vi "analyze anal files.vi"() -> ()   [LabVIEW 2024]
panel:
  out "z":cluster{dbl[], dbl[]}[](graph)=[{[-3.1923908912798504, -2.9876019813869705, -2.782813071494091, -2.578024161601211, -2.3732352517083317, -2.1684463418154523, -1.9636574319225724, -1.7588685220296927, -1.554079612136813, -1.3492907022439335, -1.1445017923510539, -0.9397128824581742, -0.7349239725652945, -0.5301350626724148, -0.3253461527795352, -0.12055724288665554, 0.08423166700622411, 0.28902057689910376, 0.4938094867919834, 0.698598396684863, 0.9033873065777427, 1.1081762164706224, 1.312965126363502, 1.5177540362563817, 1.7225429461492614, 1.9273318560421409, 2.1321207659350208, 2.3369096758279, 2.54169858572078, 2.7464874956136596], [9.0, 17.0, 27.0, 32.0, 37.0, 44.0, 46.0, 48.0, 62.0, 79.0, 99.0, 123.0, 154.0, 201.0, 258.0, 267.0, 252.0, 248.0, 225.0, 186.0, 138.0, 99.0, 66.0, 47.0, 34.0, 20.0, 11.0, 8.0, 4.0, 1.0]}, {array[1000 elements], array[1000 elements]}]
  out "y":cluster{dbl[], dbl[]}[](graph)=[{[-1.5308237164517153, -1.3260348065588357, -1.121245896665956, -0.9164569867730764, -0.7116680768801967, -0.506879166987317, -0.30209025709443743, -0.09730134720155777, 0.10748756269132188, 0.31227647258420155, 0.5170653824770812, 0.7218542923699608, 0.9266432022628405, 1.13143211215572, 1.3362210220485997], [0.0, 11.0, 10.0, 11.0, 9.0, 20.0, 83.0, 267.0, 252.0, 84.0, 27.0, 20.0, 17.0, 32.0, 17.0]}, {array[1000 elements], array[1000 elements]}]
  out "x":cluster{dbl[], dbl[]}[](graph)=[{[-1.8188204016021599, -1.6140314917092802, -1.4092425818164007, -1.204453671923521, -0.9996647620306414, -0.7948758521377617, -0.590086942244882, -0.3852980323520024, -0.1805091224591227, 0.024279787433756934, 0.2290686973266366, 0.4338576072195162, 0.6386465171123958, 0.8434354270052755, 1.0482243368981552, 1.2530132467910349, 1.4578021566839146, 1.6625910665767942], [18.0, 17.0, 18.0, 25.0, 36.0, 54.0, 98.0, 171.0, 230.0, 267.0, 219.0, 145.0, 83.0, 62.0, 52.0, 34.0, 33.0, 33.0]}, {array[1000 elements], array[1000 elements]}]
  in  "z length":i32=15
  in  "index (row) 2":i32=10
  in  "disabled index (col)":i32=10
  in  "index (row)":i32=10
  out "Waveform Graph":u16[][](graph)=[[119, 118, 117, 118, 125, 136, 154, 198, 271, 330, 367, 319, 245, 183, 162, 152, 134, 133, 133, 131, 0, 0, 0, 0, 0, 0, 0, 0, 0, 0], [108, 109, 105, 100, 111, 110, 111, 109, 120, 183, 367, 352, 184, 127, 120, 117, 132, 117, 132, 128, 0, 0, 0, 0, 0, 0, 0, 0, 0, 0], [109, 117, 127, 132, 137, 144, 146, 148, 162, 179, 199, 223, 254, 301, 358, 367, 352, 348, 325, 286, 238, 199, 166, 147, 134, 120, 111, 108, 104, 101]]
  out "zy size":i32[](array[numeric])=[20, 20]
  out "zx size":i32[](array[numeric])=[30, 20]
  out "yx size":i32[](array[numeric])=[20, 20]
  out "max value 2":u16=367
  out "max value":u16=367
  in  "z pos":i32
  out "zy":u16[][](graph)=[[110, 116, 111, 104, 104, 109, 105, 108, 105, 113, 109, 120, 116, 109, 109, 112, 114, 113, 109, 109], [105, 112, 115, 108, 105, 106, 107, 112, 111, 114, 117, 123, 118, 115, 112, 111, 111, 115, 108, 113], [105, 111, 116, 113, 112, 109, 109, 115, 113, 118, 127, 128, 117, 119, 119, 118, 115, 122, 112, 118], [105, 110, 114, 112, 110, 109, 111, 112, 115, 126, 132, 135, 117, 123, 126, 126, 122, 124, 114, 119], [106, 106, 110, 109, 107, 106, 111, 112, 115, 125, 137, 143, 130, 138, 128, 130, 128, 123, 111, 109], [105, 103, 110, 113, 111, 110, 110, 108, 114, 124, 144, 147, 145, 130, 125, 128, 124, 119, 115, 117], [102, 103, 109, 114, 112, 115, 114, 111, 116, 129, 146, 154, 158, 132, 129, 130, 127, 117, 119, 123], [105, 104, 106, 110, 109, 115, 112, 114, 117, 130, 148, 161, 166, 143, 132, 124, 123, 117, 120, 126], [108, 102, 103, 108, 105, 111, 111, 113, 114, 131, 162, 179, 172, 148, 130, 125, 120, 117, 120, 123], [109, 105, 103, 106, 103, 111, 110, 110, 109, 135, 179, 199, 181, 148, 127, 125, 122, 119, 121, 120], [105, 107, 105, 103, 101, 109, 112, 108, 109, 143, 199, 226, 193, 150, 127, 121, 124, 123, 122, 124], [99, 102, 101, 100, 101, 108, 113, 112, 113, 145, 223, 268, 210, 145, 120, 118, 121, 125, 121, 120], [100, 108, 112, 104, 100, 114, 116, 106, 112, 149, 254, 293, 205, 139, 118, 115, 116, 126, 122, 124], [107, 114, 117, 108, 103, 118, 111, 105, 112, 157, 301, 321, 193, 137, 120, 111, 114, 120, 126, 130], [110, 113, 107, 107, 111, 112, 113, 113, 121, 171, 358, 347, 187, 128, 122, 112, 127, 117, 137, 128], [108, 109, 105, 100, 111, 110, 111, 109, 120, 183, 367, 352, 184, 127, 120, 117, 132, 117, 132, 128], [108, 108, 107, 101, 106, 109, 109, 106, 122, 191, 352, 352, 172, 131, 118, 119, 126, 115, 123, 129], [106, 108, 107, 104, 108, 111, 108, 110, 126, 191, 348, 340, 168, 132, 120, 121, 129, 116, 119, 126], [105, 112, 103, 105, 109, 114, 108, 117, 133, 186, 325, 304, 170, 137, 121, 115, 122, 120, 116, 123], [105, 107, 103, 105, 110, 106, 108, 117, 137, 191, 286, 250, 169, 138, 129, 118, 119, 120, 113, 120], [105, 106, 104, 107, 107, 106, 107, 115, 133, 174, 238, 207, 158, 138, 131, 124, 121, 114, 113, 122], [103, 112, 107, 105, 106, 114, 107, 116, 123, 155, 199, 185, 155, 131, 130, 131, 117, 114, 116, 125], [104, 106, 103, 105, 105, 112, 104, 117, 118, 142, 166, 159, 145, 129, 134, 135, 121, 114, 117, 124], [107, 101, 98, 108, 105, 105, 100, 111, 118, 132, 147, 146, 134, 123, 132, 130, 131, 110, 115, 114], [106, 100, 98, 106, 106, 103, 101, 111, 119, 121, 134, 132, 129, 122, 133, 130, 135, 107, 111, 113], [109, 103, 100, 101, 106, 109, 107, 113, 116, 112, 120, 120, 122, 123, 132, 134, 133, 108, 109, 112], [106, 103, 102, 101, 104, 110, 108, 110, 110, 107, 111, 113, 110, 119, 124, 138, 127, 103, 111, 108], [101, 103, 103, 100, 103, 106, 104, 107, 104, 108, 108, 110, 111, 116, 116, 140, 122, 107, 111, 108], [103, 102, 105, 104, 106, 107, 107, 104, 101, 113, 104, 113, 112, 115, 121, 133, 111, 115, 117, 118], [108, 105, 109, 101, 106, 108, 109, 107, 102, 113, 101, 118, 112, 119, 128, 135, 114, 115, 122, 115]]
  out "zx":u16[][](graph)=[[123, 116, 111, 112, 115, 108, 108, 120, 114, 105, 109, 118, 111, 108, 105, 111, 113, 115, 114, 111], [116, 112, 111, 116, 119, 113, 110, 117, 117, 115, 117, 116, 111, 107, 106, 111, 116, 117, 115, 113], [112, 110, 113, 122, 122, 115, 115, 119, 119, 123, 127, 123, 120, 109, 111, 117, 117, 116, 116, 116], [113, 115, 120, 122, 116, 115, 118, 123, 122, 128, 132, 126, 120, 115, 115, 121, 118, 116, 119, 116], [115, 122, 119, 117, 119, 121, 125, 129, 132, 134, 137, 135, 124, 121, 121, 120, 115, 112, 114, 111], [112, 114, 107, 115, 124, 130, 131, 135, 140, 141, 144, 139, 129, 124, 123, 119, 111, 109, 110, 111], [106, 106, 115, 122, 131, 137, 139, 147, 159, 153, 146, 138, 131, 127, 123, 116, 116, 117, 114, 116], [102, 107, 119, 127, 132, 143, 154, 174, 168, 159, 148, 143, 138, 133, 126, 117, 119, 123, 123, 119], [107, 113, 123, 130, 136, 147, 175, 181, 174, 168, 162, 156, 149, 139, 131, 124, 122, 123, 123, 122], [110, 116, 123, 131, 136, 145, 179, 193, 186, 182, 179, 166, 150, 142, 130, 124, 123, 118, 119, 120], [110, 113, 116, 121, 126, 157, 190, 215, 213, 209, 199, 168, 156, 143, 129, 126, 125, 119, 118, 117], [111, 108, 109, 114, 129, 153, 191, 222, 236, 238, 223, 191, 161, 145, 136, 131, 130, 122, 118, 118], [109, 106, 104, 114, 129, 151, 186, 224, 247, 263, 254, 218, 175, 156, 142, 133, 123, 125, 123, 125], [109, 107, 107, 113, 129, 150, 182, 226, 254, 294, 301, 259, 204, 168, 148, 130, 126, 124, 124, 127], [113, 114, 114, 119, 130, 145, 172, 211, 277, 332, 358, 298, 228, 179, 147, 141, 132, 124, 127, 129], [119, 118, 117, 118, 125, 136, 154, 198, 271, 330, 367, 319, 245, 183, 162, 152, 134, 133, 133, 131], [115, 115, 114, 114, 117, 125, 145, 184, 267, 330, 352, 325, 265, 198, 166, 150, 140, 138, 136, 130], [113, 112, 112, 111, 112, 115, 139, 180, 247, 314, 348, 340, 280, 205, 156, 142, 136, 135, 133, 135], [115, 113, 111, 108, 107, 113, 135, 164, 211, 282, 325, 333, 290, 200, 156, 140, 134, 133, 133, 134], [116, 113, 107, 104, 106, 114, 124, 146, 184, 242, 286, 314, 291, 213, 160, 141, 136, 133, 130, 124], [115, 112, 111, 107, 112, 115, 120, 133, 163, 199, 238, 293, 275, 220, 164, 140, 133, 127, 119, 126], [118, 118, 114, 108, 113, 116, 116, 124, 139, 164, 199, 230, 244, 210, 171, 146, 134, 123, 123, 130], [124, 120, 113, 112, 114, 113, 108, 112, 124, 146, 166, 190, 203, 202, 176, 149, 132, 127, 126, 131], [127, 117, 111, 111, 110, 105, 109, 110, 118, 132, 147, 164, 179, 186, 171, 136, 127, 127, 124, 124], [119, 118, 110, 109, 104, 109, 113, 115, 116, 123, 134, 145, 155, 168, 165, 138, 128, 125, 118, 118], [114, 113, 112, 112, 110, 111, 113, 111, 110, 114, 120, 125, 132, 153, 155, 145, 131, 126, 116, 115], [114, 114, 116, 116, 112, 109, 108, 107, 105, 106, 111, 116, 125, 131, 144, 143, 133, 121, 115, 125], [114, 118, 117, 115, 110, 108, 107, 106, 105, 105, 108, 112, 116, 123, 136, 141, 125, 116, 125, 123], [117, 114, 113, 111, 109, 112, 110, 108, 108, 105, 104, 106, 111, 119, 132, 131, 118, 120, 119, 123], [114, 110, 109, 108, 108, 113, 113, 112, 113, 108, 101, 104, 109, 115, 121, 122, 125, 119, 118, 121]]
  in  "max":dbl
  in  "x pos":i32=15
  in  "xy length":i32=10
  in  "y pos":i32=15
  in  "color 2":T1={"color array"=[0, 16448250, 16776281, 16448250, 16776960, 16711680, 16448250, 16448250], "num of colors"=2, "max"=369.6999999999998, "min"=100.0} {"min" step=0.01 format="%_2f"; "max" step=0.1 format="%_3f"}
  out "input cluster":T2={"x profile"=[[127.98499244810402, 128.01819992638715, 128.27479837597622, 129.75131149476877, 136.03985950741094, 155.66612894300334, 199.74424439891834, 268.3361808480487, 335.10154662409263, 358.5949867435007, 321.7194030139125, 250.78530549712218, 186.71372418795545, 149.17529291854723, 133.75194927458324, 129.1669569612915, 128.16527498857147, 128.00302210343048], [118.0, 117.0, 118.0, 125.0, 136.0, 154.0, 198.0, 271.0, 330.0, 367.0, 319.0, 245.0, 183.0, 162.0, 152.0, 134.0, 133.0, 133.0]], "y profile"=[[114.70284653862177, 114.70284653954327, 114.702848277479, 114.70377495170128, 114.84312668808873, 120.70115602787637, 187.28656278735298, 363.2605402152609, 355.57849742616287, 180.76249711116822, 119.82977577612944, 114.81545111852968, 114.70354643293737, 114.70284776970243, 114.70284653923443], [100.0, 111.0, 110.0, 111.0, 109.0, 120.0, 183.0, 367.0, 352.0, 184.0, 127.0, 120.0, 117.0, 132.0, 117.0]], "z profile"=[[119.55704773743344, 119.61939358824723, 119.78974190490983, 120.21997532872496, 121.22357109757961, 123.38362009431867, 127.66767738146085, 135.48383601701704, 148.57195700374172, 168.62168507268728, 196.58875195778302, 231.85404323967833, 271.57160270784686, 310.64386394428163, 342.61097740956944, 361.3397167221943, 362.933006958581, 347.04975953745355, 317.0236767601359, 278.72445092692647, 238.69338325035702, 202.36176800094552, 172.99730410880292, 151.57887205021876, 137.3686141967263, 128.74959458071595, 123.95396358981732, 121.50024581938149, 120.34367079281783, 119.84076858586502], [109.0, 117.0, 127.0, 132.0, 137.0, 144.0, 146.0, 148.0, 162.0, 179.0, 199.0, 223.0, 254.0, 301.0, 358.0, 367.0, 352.0, 348.0, 325.0, 286.0, 238.0, 199.0, 166.0, 147.0, 134.0, 120.0, 111.0, 108.0, 104.0, 101.0]], "FWHMx[um]"=0.9086257593875379, "FWHMy[um]"=0.429218030475882, "FWHMz[um]"=1.7721806371618676, "z pos"=16, "tilt"=0.0, "error x"=0.2602998640251688, "error y"=0.17305857039380643, "error z"=0.5303895340703632, "error max"=0.5303895340703632, "coeffs x"=[231.07045695661935, 8.881439930285008, 1.8841734793030511, 60.14760852604164, 127.98153349634119], "coeffs y"=[286.6205920264443, 7.475129963104222, 0.8900487593555202, 49.60214990152288, 114.70284653862163], "coeffs z"=[244.93564609838174, 15.588690290649607, 3.6748856419451528, 129.91130321134406, 119.52673189791437], "profiles x"=[{[-1.8188204016021599, -1.6140314917092802, -1.4092425818164007, -1.204453671923521, -0.9996647620306414, -0.7948758521377617, -0.590086942244882, -0.3852980323520024, -0.1805091224591227, 0.024279787433756934, 0.2290686973266366, 0.4338576072195162, 0.6386465171123958, 0.8434354270052755, 1.0482243368981552, 1.2530132467910349, 1.4578021566839146, 1.6625910665767942], [18.0, 17.0, 18.0, 25.0, 36.0, 54.0, 98.0, 171.0, 230.0, 267.0, 219.0, 145.0, 83.0, 62.0, 52.0, 34.0, 33.0, 33.0]}, {array[1000 elements], array[1000 elements]}], "profiles y"=[{[-1.5308237164517153, -1.3260348065588357, -1.121245896665956, -0.9164569867730764, -0.7116680768801967, -0.506879166987317, -0.30209025709443743, -0.09730134720155777, 0.10748756269132188, 0.31227647258420155, 0.5170653824770812, 0.7218542923699608, 0.9266432022628405, 1.13143211215572, 1.3362210220485997], [0.0, 11.0, 10.0, 11.0, 9.0, 20.0, 83.0, 267.0, 252.0, 84.0, 27.0, 20.0, 17.0, 32.0, 17.0]}, {array[1000 elements], array[1000 elements]}], "profiles z"=[{[-3.1923908912798504, -2.9876019813869705, -2.782813071494091, -2.578024161601211, -2.3732352517083317, -2.1684463418154523, -1.9636574319225724, -1.7588685220296927, -1.554079612136813, -1.3492907022439335, -1.1445017923510539, -0.9397128824581742, -0.7349239725652945, -0.5301350626724148, -0.3253461527795352, -0.12055724288665554, 0.08423166700622411, 0.28902057689910376, 0.4938094867919834, 0.698598396684863, 0.9033873065777427, 1.1081762164706224, 1.312965126363502, 1.5177540362563817, 1.7225429461492614, 1.9273318560421409, 2.1321207659350208, 2.3369096758279, 2.54169858572078, 2.7464874956136596], [9.0, 17.0, 27.0, 32.0, 37.0, 44.0, 46.0, 48.0, 62.0, 79.0, 99.0, 123.0, 154.0, 201.0, 258.0, 267.0, 252.0, 248.0, 225.0, 186.0, 138.0, 99.0, 66.0, 47.0, 34.0, 20.0, 11.0, 8.0, 4.0, 1.0]}, {array[1000 elements], array[1000 elements]}], "x pos"=57, "y pos"=29}
  out "yx":u16[][](graph)=[[107, 103, 102, 103, 101, 99, 97, 99, 106, 106, 108, 111, 110, 111, 113, 110, 103, 105, 105, 105], [105, 100, 99, 102, 105, 104, 100, 98, 98, 103, 109, 115, 118, 115, 111, 109, 108, 112, 107, 102], [106, 107, 105, 107, 107, 105, 106, 107, 108, 105, 105, 107, 110, 111, 110, 109, 111, 112, 109, 106], [99, 98, 100, 105, 104, 102, 109, 107, 102, 99, 100, 104, 107, 113, 114, 115, 110, 109, 111, 114], [102, 102, 105, 106, 106, 106, 108, 108, 102, 105, 111, 110, 112, 114, 119, 125, 122, 116, 113, 114], [107, 110, 111, 112, 115, 115, 112, 116, 113, 113, 110, 113, 117, 118, 126, 132, 121, 126, 124, 121], [112, 113, 109, 108, 111, 112, 118, 116, 107, 103, 111, 113, 113, 119, 129, 128, 130, 141, 142, 136], [101, 100, 101, 104, 107, 112, 117, 119, 114, 109, 109, 109, 113, 122, 127, 129, 132, 143, 148, 145], [103, 99, 104, 110, 115, 121, 129, 135, 135, 123, 120, 119, 119, 123, 123, 132, 158, 159, 152, 152], [110, 106, 106, 113, 122, 134, 152, 176, 192, 188, 183, 170, 152, 135, 133, 134, 140, 151, 149, 144], [119, 118, 117, 118, 125, 136, 154, 198, 271, 330, 367, 319, 245, 183, 162, 152, 134, 133, 133, 131], [116, 121, 126, 123, 121, 123, 137, 173, 219, 287, 352, 344, 282, 220, 189, 168, 135, 128, 126, 122], [123, 126, 128, 124, 121, 118, 120, 133, 142, 161, 184, 193, 184, 157, 152, 145, 128, 121, 120, 123], [133, 130, 133, 138, 134, 127, 122, 122, 123, 125, 127, 130, 124, 120, 120, 122, 117, 123, 123, 123], [138, 133, 135, 141, 143, 137, 126, 117, 117, 117, 120, 121, 118, 120, 119, 122, 114, 114, 114, 113], [141, 144, 145, 145, 146, 142, 127, 117, 124, 124, 117, 115, 110, 104, 104, 109, 114, 112, 105, 103], [134, 141, 145, 148, 149, 146, 130, 131, 133, 134, 132, 120, 117, 113, 109, 109, 115, 114, 117, 118], [129, 134, 135, 139, 141, 141, 138, 132, 134, 123, 117, 115, 114, 110, 109, 112, 116, 112, 110, 113], [118, 123, 124, 123, 130, 133, 140, 129, 127, 135, 132, 127, 123, 119, 117, 115, 110, 112, 111, 112], [129, 127, 124, 127, 132, 135, 141, 136, 133, 135, 128, 125, 122, 118, 120, 117, 114, 113, 118, 120]]
  out "r or z":dbl=7.0
  out "String":string="E:\\20241006-205850beads\\20241006-205850beadsaiviatif\\20241006-205850beads_t0.aivia.tif"
  in  "index":i32=56
  in  "stop":bool
  out "Numeric":i32=84
  in  "file path (use dialog)":path=path "E:/PSFvsR.anal"
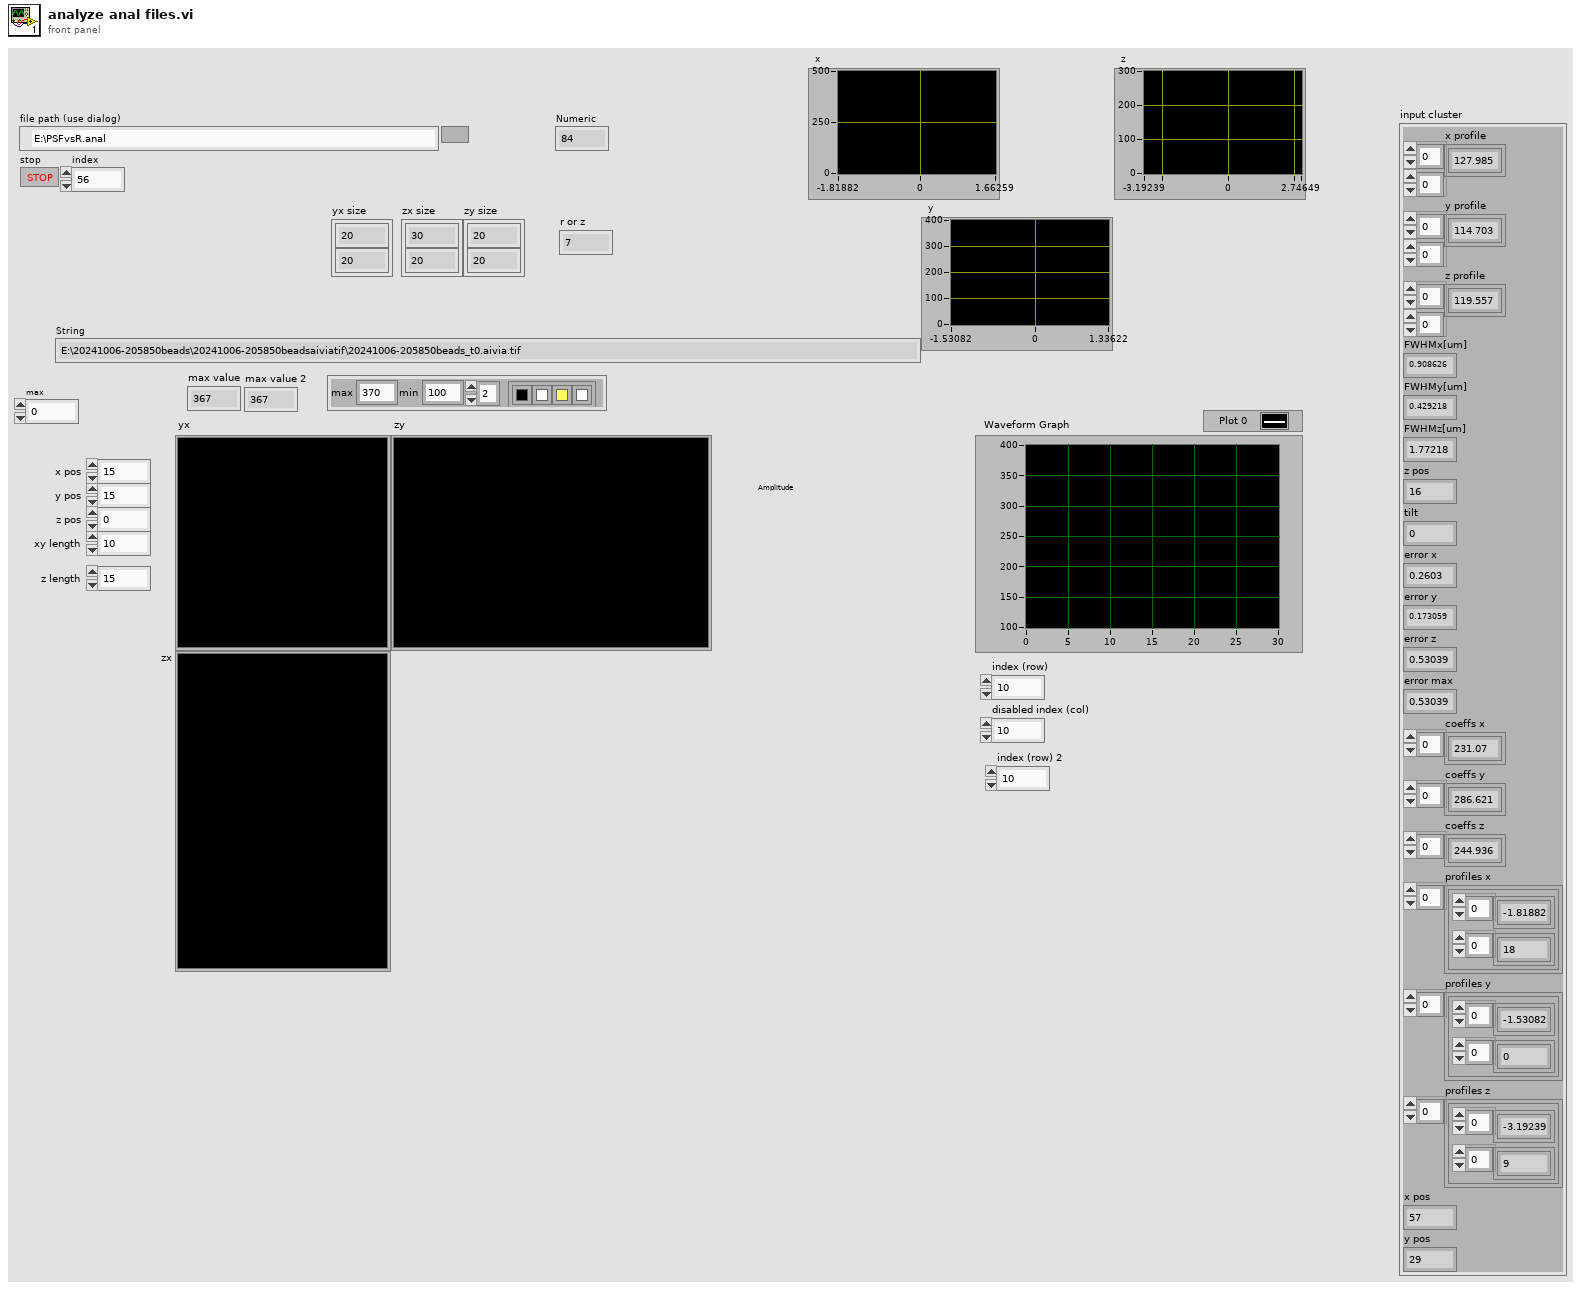
[diagram p1: front panel]
types:
  T1 = cluster{"color array":u32[], "num of colors":i32, "max":dbl, "min":dbl}
  T2 = cluster{"x profile":dbl[][], "y profile":dbl[][], "z profile":dbl[][], "FWHMx[um]":dbl, "FWHMy[um]":dbl, "FWHMz[um]":dbl, "z pos":i32, "tilt":dbl, "error x":dbl, "error y":dbl, "error z":dbl, "error max":dbl, "coeffs x":dbl[], "coeffs y":dbl[], "coeffs z":dbl[], "profiles x":cluster{dbl[], dbl[]}[], "profiles y":cluster{dbl[], dbl[]}[], "profiles z":cluster{dbl[], dbl[]}[], "x pos":i32, "y pos":i32}
  T3 = cluster{"z [um]":dbl, "Particle Report":cluster{"Area":dbl, "Number of Holes":dbl, "Bounding Rect":cluster{"Left":dbl, "Top":dbl, "Right":dbl, "Bottom":dbl}, "Center of Mass":cluster{"X":dbl, "Y":dbl}, "Orientation":dbl, "Dimensions":cluster{"Width":dbl, "Height":dbl}}, "yx":u16[][], "zx":u16[][], "zy":u16[][], "filepath":string, "FWHMx'":dbl, "x' profiles":cluster{"fit x":dbl[], "fit y":dbl[]}[], "FWHMz'":dbl, "z' profiles":cluster{"fit x":dbl[], "fit y":dbl[]}[], "input cluster":cluster{"x profile":dbl[][], "y profile":dbl[][], "z profile":dbl[][], "FWHMx[um]":dbl, "FWHMy[um]":dbl, "FWHMz[um]":dbl, "z pos":i32, "tilt":dbl, "error x":dbl, "error y":dbl, "error z":dbl, "error max":dbl, "coeffs x":dbl[], "coeffs y":dbl[], "coeffs z":dbl[], "profiles x":cluster{dbl[], dbl[]}[], "profiles y":cluster{dbl[], dbl[]}[], "profiles z":cluster{dbl[], dbl[]}[], "x pos":i32, "y pos":i32}}
  T4 = cluster{"Area":dbl, "Number of Holes":dbl, "Bounding Rect":cluster{"Left":dbl, "Top":dbl, "Right":dbl, "Bottom":dbl}, "Center of Mass":cluster{"X":dbl, "Y":dbl}, "Orientation":dbl, "Dimensions":cluster{"Width":dbl, "Height":dbl}}
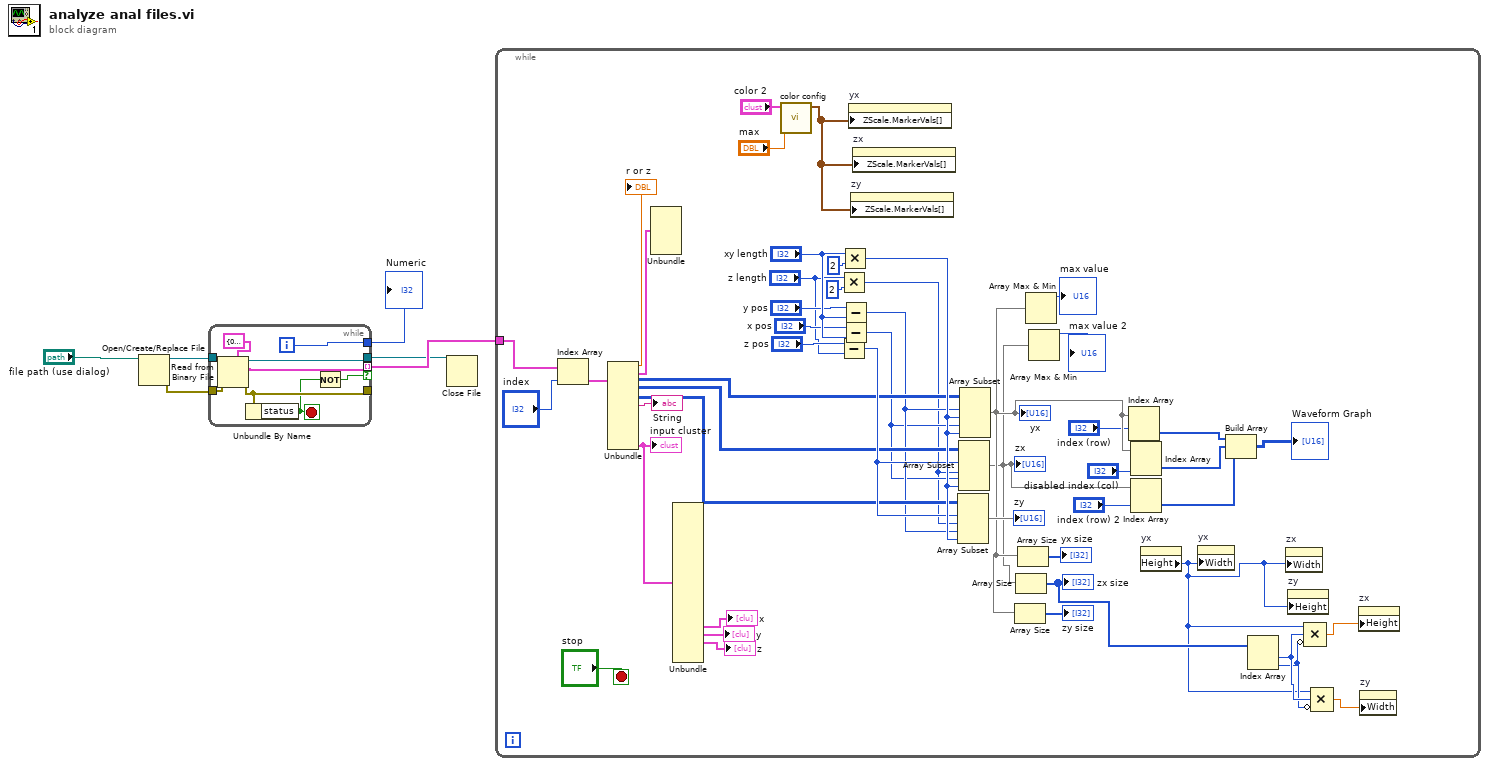
[diagram p0: block diagram]
diagram:
  n1 = Open/Create/Replace File(file path (use dialog)="file path (use dialog)") -> (refnum out=w5:refnum<file>, error out=w4:errorcluster)  [unwired: 5 in, 1 out]
  n2 = while {
    tunnel: w5 -> [w15]
    tunnel: w4 -> [w14]
    tunnel: [w13] -> w2 mode=indexing if=w8
    tunnel: [w12] -> w1
    tunnel: [w10] -> _
    tunnel: [w11] -> w3
    i -> [w11]
    stop <- w7 stop-if-true
    n3 = Read from Binary File(5:T3 {"z [um]"=0.0, "Particle Report"={"Area"=0.0, "Number of Holes"=0.0, "Bounding Rect"={"Left"=0.0, "Top"=0.0, "Right"=0.0, "Bottom"=0.0}, "Center of Mass"={"X"=0.0, "Y"=0.0}, "Orientation"=0.0, "Dimensions"={"Width"=0.0, "Height"=0.0}}, "yx"=[], "zx"=[], "zy"=[], "filepath"="", "FWHMx'"=0.0, "x' profiles"=[], "FWHMz'"=0.0, "z' profiles"=[], "input cluster"={"x profile"=[], "y profile"=[], "z profile"=[], "FWHMx[um]"=0.0, "FWHMy[um]"=0.0, "FWHMz[um]"=0.0, "z pos"=0, "tilt"=0.0, "error x"=0.0, "error y"=0.0, "error z"=0.0, "error max"=0.0, "coeffs x"=[375.1262519235072, 15.692898037016759, 2.741983029822066, 316.1979872885655, 113.96523182291966], "coeffs y"=[375.1262519235072, 15.692898037016759, 2.741983029822066, 316.1979872885655, 113.96523182291966], "coeffs z"=[375.1262519235072, 15.692898037016759, 2.741983029822066, 316.1979872885655, 113.96523182291966], "profiles x"=[], "profiles y"=[], "profiles z"=[], "x pos"=0, "y pos"=0}} ("output cluster"), 8:w14, 11:w15) -> (0:w10:errorcluster, 2:w13:T3, 3:w12:refnum<file>)  [unwired: 3 in, 1 out]
    n4 = Unbundle By Name(w10) -> ("status"=w7:bool)
    n5 = Not(x=w7) -> (.not. x?=w8:bool)
  }
  "Numeric" <- w3
  n6 = Close File(refnum=w1) -> ()  [unwired: 1 in, 2 out]
  n7 = while {
    tunnel: w2 -> [w59]
    stop <- "stop" stop-if-true
    n8 = Index Array(array=w59, index="index") -> (element=w62:T3)
    n9 = Unbundle(w62) -> ("z [um]"=→"r or z":dbl, "Particle Report"=w61:T4, "yx"=w48:u16[][], "zx"=w47:u16[][], "zy"=w49:u16[][], "filepath"=→"String":string, "input cluster"=w19:T2)  [unwired: 4 out]
    "input cluster" <- w19
    n10 = Unbundle(w61) -> ()  [unwired: 6 out]
    n11 = Unbundle(w19) -> ("profiles x"=→"x":cluster{dbl[], dbl[]}[], "profiles y"=→"y":cluster{dbl[], dbl[]}[], "profiles z"=→"z":cluster{dbl[], dbl[]}[])  [unwired: 17 out]
    n12 = call "color config.vi"("max"="max", "color 1"="color 2") -> ("Array"=w54:cluster{dbl, u32}[])  [unwired: 8 in, 1 out]
    n13 = Multiply(x="z length", y=2) -> (x*y=w27:i32)
    n14 = Subtract(x="z pos", y="z length") -> (x-y=w51:i32)
    n15 = Multiply(x="xy length", y=2) -> (x*y=w53:i32)
    n16 = Subtract(x="y pos", y="xy length") -> (x-y=w42:i32)
    n17 = Subtract(x="x pos", y="xy length") -> (x-y=w41:i32)
    n18 = property on="yx" class="IntGraph (strict)"("ZScale.MarkerVals[]"=w54) -> ()  [unwired: 2 in, 2 out]
    n19 = property on="zy" class="IntGraph (strict)"("ZScale.MarkerVals[]"=w54) -> ()  [unwired: 2 in, 2 out]
    n20 = property on="zx" class="IntGraph (strict)"("ZScale.MarkerVals[]"=w54) -> ()  [unwired: 2 in, 2 out]
    n21 = Array Subset(array=w49, index (row)=w51, length (row)=w27, index (col)=w42, length (col)=w53) -> (→"zy":u16[][])
    n22 = Array Subset(array=w47, index (row)=w51, length (row)=w27, index (col)=w41, length (col)=w53) -> (w39:u16[][])
    "zx" <- w39
    n23 = Array Subset(array=w48, index (row)=w42, length (row)=w53, index (col)=w41, length (col)=w53) -> (w40:u16[][])
    "yx" <- w40
    n24 = Array Size(array=w40) -> (size(s)=→"zy size":i32[])
    n25 = Array Size(array=w39) -> (size(s)=w25:i32[])
    "zx size" <- w25
    n26 = Array Size(array=w40) -> (size(s)=→"yx size":i32[])
    n27 = Array Max & Min(array=w40) -> (max value=→"max value":u16)  [unwired: 3 out]
    n28 = Array Max & Min(array=w39) -> (max value=→"max value 2":u16)  [unwired: 3 out]
    n29 = Index Array(array=w40, index (row)="index (row)") -> (element=w35:u16[])  [unwired: 1 in]
    n30 = Index Array(array=w40, index (col)="disabled index (col)") -> (element=w34:u16[])  [unwired: 1 in]
    n31 = Index Array(array=w39, index (col)="index (row) 2") -> (element=w33:u16[])  [unwired: 1 in]
    n32 = property on="yx" class="IntGraph (strict)"() -> ("Height"=w20:u32)  [unwired: 2 in, 2 out]
    n33 = property on="yx" class="IntGraph (strict)"("Width"=w20) -> ()  [unwired: 2 in, 2 out]
    n34 = Build Array(w35, w34, w33) -> (→"Waveform Graph":u16[][])
    n35 = Index Array(array=w25) -> (element #1=w23:i32, element #2=w22:i32)  [unwired: 2 in]
    n36 = property on="zx" class="IntGraph (strict)"("Width"=w20) -> ()  [unwired: 2 in, 2 out]
    n37 = property on="zy" class="IntGraph (strict)"("Height"=w20) -> ()  [unwired: 2 in, 2 out]
    n38 = Compound Arithmetic op=MULTIPLY(w20, w23, invert w22) -> (w24:dbl)
    n39 = Compound Arithmetic op=MULTIPLY(w20, w23, invert w22) -> (w21:dbl)
    n40 = property on="zx" class="IntGraph (strict)"("Height"=w24) -> ()  [unwired: 2 in, 2 out]
    n41 = property on="zy" class="IntGraph (strict)"("Width"=w21) -> ()  [unwired: 2 in, 2 out]
  }
